vi "FindBlob_Test.vi.vi"() -> ()   [LabVIEW 2010]
panel:
  out "# particles":i32
  out "Area (pixels)":dbl[][](array[numeric]) format="%.2f"
  out "Intensity Graph 2":u8[][](graph)
  out "image":picture
  in  "Initial Image":picture caption="new picture"
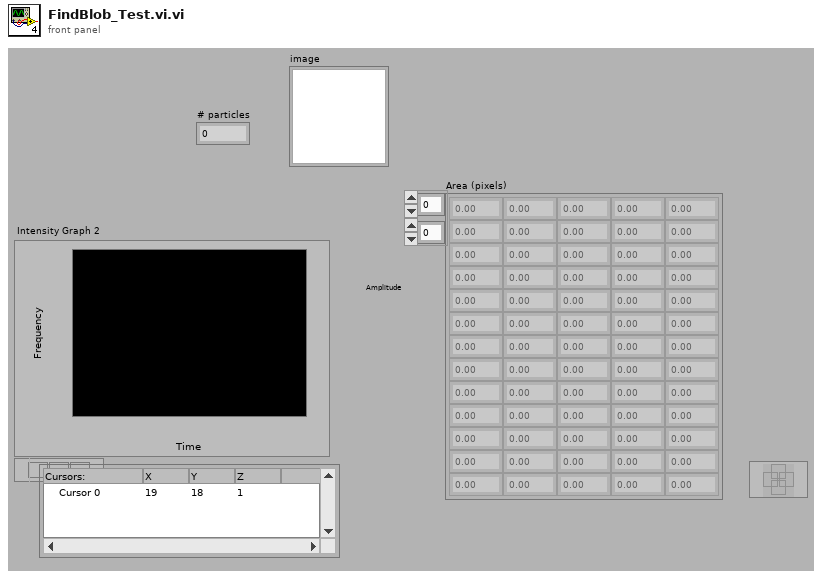
[diagram p1: front panel]
types:
  T1 = enum16{"No Change", "Apricot", "Carnation", "Ether", "Greyscale", "Greyscale-banded", "Hot Metal", "Lava Waves", "Mac", "Morning Glory", "Rainbow", "Rainbow-banded", "Rainbow-inverted", "Rainbow-striped", "Saturn", "Seismic", "Space"}
  T2 = typedef "QT_Image.ctl" = cluster{"Width":i32, "Height":i32, "Depth":i32, "data":u8[], "Compressed data":u8[], "Color table":u32[], "Duration":i32, "Options":i32, "Timestamp":i32, "ID":i32, "Reserved":i32, "Dialogs":u32}
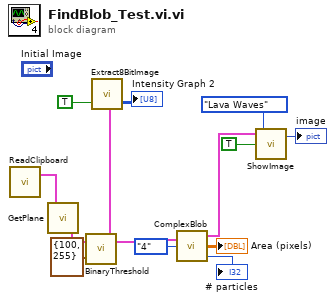
[diagram p0: block diagram]
diagram:
  n1 = call <userlib>:"ReadClipboard.vi"() -> ("Image Out"=w10:T2)  [unwired: 3 out]
  n2 = call <userlib>:"GetPlane.vi"("Image In"=w10) -> ("Greyscale  Out"=w12:T2)  [unwired: 3 out]
  n3 = call <userlib>:"BinaryThreshold.vi"("threshold"=cluster{u8, u8} {100, 255}, "Image In"=w12) -> ("Image Out"=w7:T2)  [unwired: 1 out]
  n4 = call <userlib>:"Extract8BitImage.vi"("Flip?"=TRUE, "Image in"=w7) -> ("Intensity Graph"=→"Intensity Graph 2":u8[][])  [unwired: 1 out]
  n5 = call <userlib>:"ComplexBlob.vi"("Connectivity"=enum16{"4", "8"}."4", "Image in"=w7) -> ("# particles"=→"# particles":i32, "Parameters"=→"Area (pixels)":dbl[][], "Image out"=w6:T2)  [unwired: 1 out]
  n6 = call <userlib>:"ShowImage.vi"("Color Table"=T1."Lava Waves", "Autoscale?"=TRUE, "Image"=w6) -> ("image"=→"image":picture)  [unwired: 1 out]
